vi "Concatenar por Cursor.vi"(8 "error in":errorcluster, 10 "Cluster 3":T1, 11 "WaveformGraph in":refnum<vi>) -> (0 "error out":errorcluster, 2 "output cluster":T1)   [LabVIEW 2020]
uses:
  Dados consumidor.ctl
  <vilib>/Waveform/WDTOps.llb/WDT Waveform Duration DBL.vi
  <vilib>/Waveform/WDTOps.llb/WDT Get Waveform Subset DBL.vi
  <vilib>/Waveform/WDTOps.llb/WDT Append Waveforms DBL.vi
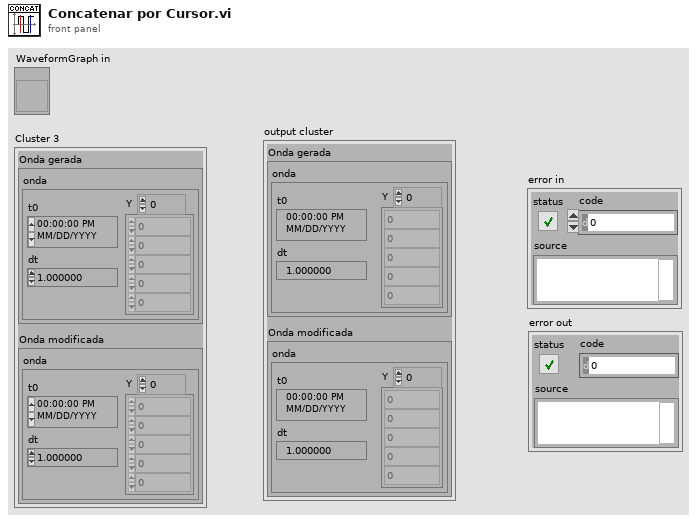
[diagram p1: front panel]
types:
  T1 = typedef "Dados consumidor.ctl" = cluster{"Onda gerada":cluster{"onda":waveform(dbl)}, "Onda modificada":cluster{"onda":waveform(dbl)}}
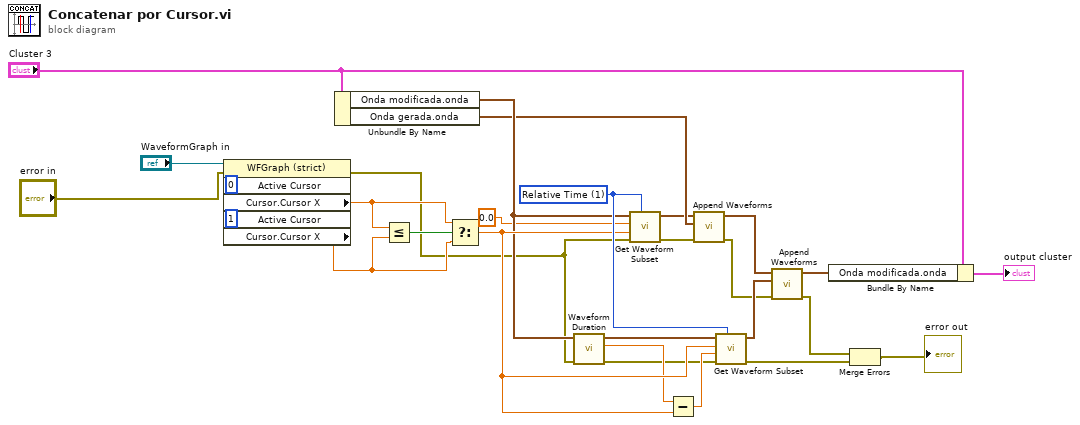
[diagram p0: block diagram]
diagram:
  w26 = u16 1 items=["Samples", "Relative Time"] ("start/duration format")
  n1 = property on="Property Node" class="WFGraph (strict)"(reference="WaveformGraph in", error in="error in", "Active Cursor"=u32 0, "Active Cursor"=u32 1) -> (error out=w7:errorcluster, "Cursor.Cursor X"=w13:dbl, "Cursor.Cursor X"=w19:dbl)  [unwired: 1 out]
  n2 = Unbundle By Name("Cluster 3") -> ("Onda modificada.onda"=w20:waveform(dbl), "Onda gerada.onda"=w17:waveform(dbl))
  n3 = Less Or Equal?(x=w13, y=w19) -> (x <= y?=w12:bool)
  n4 = Select(t=w13, s=w12, f=w19) -> (s? t:f=w24:dbl)
  n5 = call-poly <vilib>:"Waveform Duration.vi"("error in (no error)"=w7, "waveform in"=w20) -> ("error out"=w6:errorcluster, "duration"=w22:dbl, "waveform out"=w21:waveform(dbl))  [unwired: 7 in]
  n6 = call-poly <vilib>:"Get Waveform Subset.vi"("start/duration format"=w26, "error in (no error)"=w7, "duration"=w24, "start samples/time"=0.0, "waveform in"=w20) -> ("error out"=w5:errorcluster, "waveform out"=w15:waveform(dbl))  [unwired: 1 in, 2 out]
  n7 = Subtract(x=w22, y=w24) -> (x-y=w23:dbl)
  n8 = call-poly <vilib>:"Append Waveforms.vi"("error in (no error)"=w5, "waveform B"=w17, "waveform A"=w15) -> ("error out"=w4:errorcluster, "waveform out"=w16:waveform(dbl))  [unwired: 7 in]
  n9 = call-poly <vilib>:"Get Waveform Subset.vi"("start/duration format"=w26, "error in (no error)"=w6, "duration"=w23, "start samples/time"=w24, "waveform in"=w21) -> ("error out"=w2:errorcluster, "waveform out"=w25:waveform(dbl))  [unwired: 1 in, 2 out]
  n10 = call-poly <vilib>:"Append Waveforms.vi"("error in (no error)"=w4, "waveform B"=w25, "waveform A"=w16) -> ("error out"=w3:errorcluster, "waveform out"=w27:waveform(dbl))  [unwired: 7 in]
  n11 = Bundle By Name(cluster="Cluster 3", "Onda modificada.onda"=w27) -> (→"output cluster":T1)
  n12 = Merge Errors(w3, w2) -> (→"error out":errorcluster)
